vi "Configure Action Core.vi"(8 "error in (no error)":errorcluster, 11 "NI DMM in":refnum<class "NI DMM.lvclass">) -> (0 "error out":errorcluster, 3 "NI DMM out":refnum<class "NI DMM.lvclass">)   [LabVIEW 2020, in "NI DMM.lvlib" / "NI DMM.lvclass"]
uses:
  NI DMM.lvclass
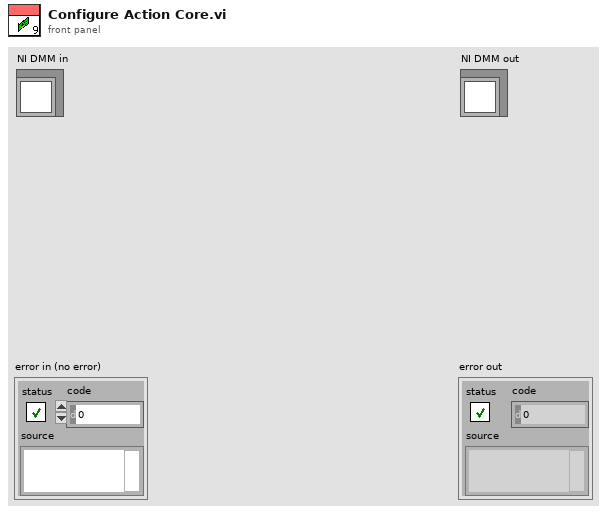
[diagram p1: front panel]
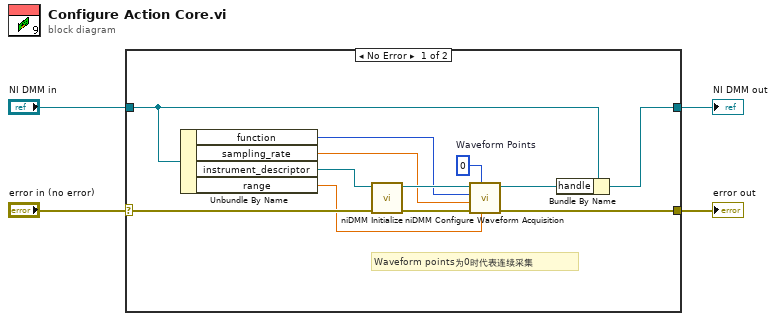
[diagram p0: block diagram]
diagram:
  n1 = case shown="No Error" "error in (no error)" {
    selector: "error in (no error)" -> [w16 w18]
    tunnel: [w6 w18] -> w3
    tunnel: "NI DMM in" -> [w8 w17]
    tunnel: [w5 w17] -> w1
    frame No Error {
      w13 = 0  # Waveform Points
      # "Waveform points为0时代表连续采集"
      n2 = Unbundle By Name(w8) -> ("function"=w9:i32, "sampling_rate"=w10:dbl, "instrument_descriptor"=w12:refnum<k15>, "range"=w11:dbl)
      n3 = call <instrlib>:"niDMM Initialize.vi"("error in (no error)"=w16, "Instrument Descriptor"=w12) -> ("error out"=w15:errorcluster, "instrument handle out"=w14:refnum<k15>)  [unwired: 8 in]
      n4 = call <instrlib>:"niDMM Configure Waveform Acquisition.vi"("Range"=w11, "Waveform Points"=w13, "error in (no error)"=w15, "Rate"=w10, "Function"=w9, "instrument handle"=w14) -> ("error out"=w6:errorcluster, "instrument handle out"=w7:refnum<k15>)  [unwired: 4 in]
      n5 = Bundle By Name(cluster=w8, "handle"=w7) -> (w5:refnum<class "NI DMM.lvclass">)
    }
    frame Error {
    }
  }
  "error out" <- w3
  "NI DMM out" <- w1
